vi "Inline Replace Core.vi"(7 "Prevent Overwrite? (F)":bool, 8 "error in (no error)":errorcluster, 9 "renamed keys":string[](array[string]), 10 "keys":string[](array[string]), 11 "Variant in":variant) -> (0 "error out":errorcluster, 1 "replaced?":bool[](array[boolean]), 2 "Found?":bool[](array[boolean]), 3 "Variant out":variant)   [LabVIEW 2023, in "uData.lvlib" / "uData.lvclass"]
uses:
  uData.lvclass
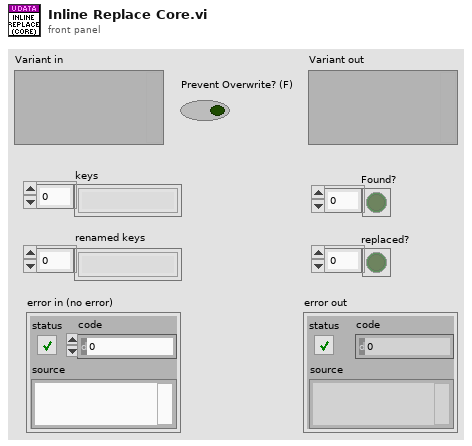
[diagram p1: front panel]
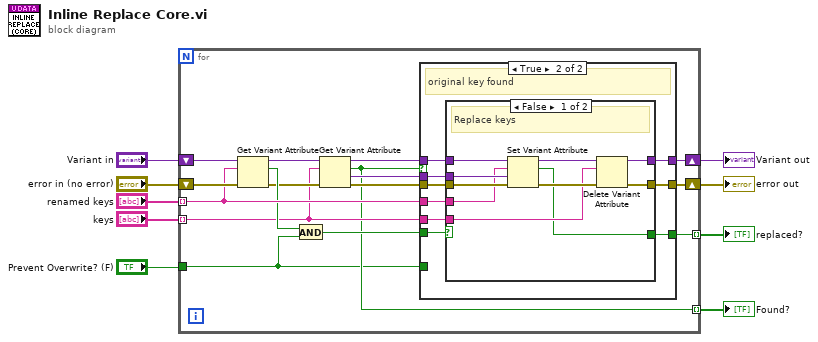
[diagram p0: block diagram]
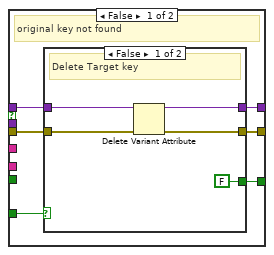
[diagram p2: hidden frame]
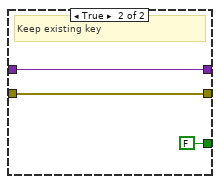
[diagram p3: hidden frame]
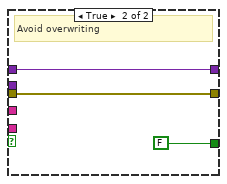
[diagram p4: hidden frame]
diagram:
  n1 = for {
    tunnel: "renamed keys" -> [w21] mode=indexing
    tunnel: "keys" -> [w13] mode=indexing
    shift-right: [w25] -> w9
    shift-left: "Variant in" -> [w23]
    shift-right: [w24] -> w7
    shift-left: "error in (no error)" -> [w22]
    tunnel: [w11] -> w3 mode=indexing
    tunnel: "Prevent Overwrite? (F)" -> [w10]
    tunnel: [w18] -> w1 mode=indexing
    n2 = Get Variant Attribute(Variant=w23, name=w21, error in=w22) -> (duplicate Variant=w15:variant, found=w20:bool, error out=w17:errorcluster)  [unwired: 1 in, 1 out]
    n3 = And(x=w20, y=w10) -> (x .and. y?=w19:bool)
    n4 = Get Variant Attribute(Variant=w15, name=w13, error in=w17) -> (duplicate Variant=w14:variant, found=w11:bool, value=w12:variant, error out=w16:errorcluster)  [unwired: 1 in]
    n5 = case shown="True" w11 {
      tunnel: [w29 w48] -> w25
      tunnel: [w27 w47] -> w24
      tunnel: w21 -> [_ w46]
      tunnel: w19 -> [_ w45]
      tunnel: [w31 w44] -> w18
      tunnel: w16 -> [w28 w43]
      tunnel: w14 -> [w30 w42]
      tunnel: w13 -> [_ w41]
      tunnel: w12 -> [_ w40]
      tunnel: w10 -> [w26 _]
      frame False {
        # "original key not found"
        n6 = case shown="False" w26 {
          tunnel: [FALSE ("replaced") FALSE ("replaced")] -> w31
          tunnel: w30 -> [w35 w39]
          tunnel: [w33 w39] -> w29
          tunnel: w28 -> [w34 w38]
          tunnel: [w32 w38] -> w27
          frame False {
            # "Delete Target key"
            n7 = Delete Variant Attribute(4:w34, 7:w35) -> (0:w32:errorcluster, 3:w33:variant)  [unwired: 1 in, 1 out]
          }
          frame True {
            # "Keep existing key"
          }
        }
      }
      frame True {
        # "original key found"
        n8 = case shown="False" w45 {
          tunnel: [w51 w61] -> w48
          tunnel: [w53 w59] -> w47
          tunnel: w41 -> [w50 _]
          tunnel: w42 -> [w57 w61]
          tunnel: w43 -> [w56 w59]
          tunnel: w46 -> [w54 _]
          tunnel: [w49 FALSE] -> w44
          tunnel: w40 -> [w55 _]
          frame False {
            # "Replace keys"
            n9 = Set Variant Attribute(Variant=w57, name=w54, value=w55, error in=w56) -> (Variant out=w52:variant, replaced=w49:bool, error out=w58:errorcluster)
            n10 = Delete Variant Attribute(4:w58, 6:w50, 7:w52) -> (0:w53:errorcluster, 3:w51:variant)  [unwired: 1 out]
          }
          frame True {
            # "Avoid overwriting"
          }
        }
      }
    }
  }
  "error out" <- w7
  "Variant out" <- w9
  "replaced?" <- w1
  "Found?" <- w3
